vi "FGV_DAQ_DI_Task.vi"(3 "error in":errorcluster, 4 "DI task":refnum<k21>, 5 "Action":T1) -> (0 "error out":errorcluster, 1 "DI task":refnum<k21>)   [LabVIEW 2026]
uses:
  Controls/TypeDef_FGV.ctl
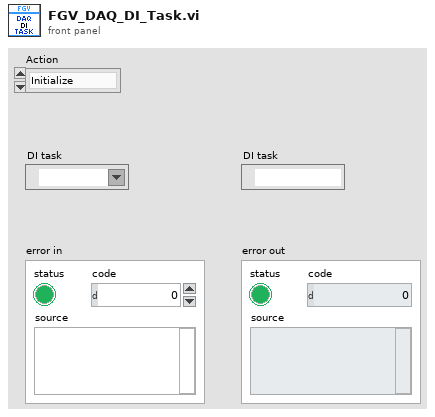
[diagram p1: front panel]
types:
  T1 = typedef "TypeDef_FGV.ctl" = enum16{"Initialize", "Write", "Read"}
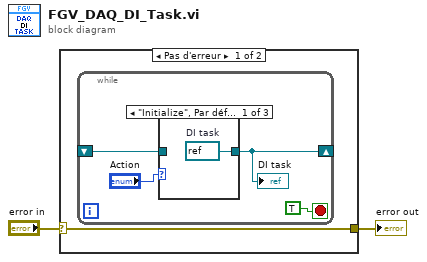
[diagram p0: block diagram]
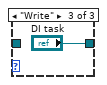
[diagram p3: hidden frame]
diagram:
  n1 = case shown="Pas d'erreur" "error in" {
    selector: "error in" -> [w3 w11]
    tunnel: [w3 w11] -> w2
    frame No Error {
      n2 = while {
        shift-right: [w4] -> _
        shift-left: _ -> [w5]
        stop <- TRUE stop-if-true
        n3 = case shown="\"Initialize\", Par défaut" "Action" {
          tunnel: [w8 w9 "DI task"] -> w4
          tunnel: w5 -> [_ w9 _]
          frame "Initialize", Default {
            w8 = refnum<k21> refnum  # DI task
          }
          frame "Read" {
          }
          frame "Write" {
          }
        }
        "DI task" <- w4
      }
    }
    frame Error {
    }
  }
  "error out" <- w2
